vi "Attach Principal to Thing.vi"(8 "error in (no error)":errorcluster, 9 "Principal":string, 10 "Thing":string, 11 "IoT Session in":refnum<class "IoT Session.lvclass">) -> (0 "error out":errorcluster, 3 "IoT Session out":refnum<class "IoT Session.lvclass">)   [LabVIEW 2015, in "NI_AWS_IoT.lvlib" / "IoT Session.lvclass"]
uses:
  IoT Session.lvclass
  Core/HTTP Request/Request Options.ctl
  Core/HTTP Request/Name Value Pair.ctl
  Core/HTTP Request/Region handling.ctl
  Core/HTTP Request/URL formatting.ctl
  Core/HTTP Request/HTTP Request.lvclass
panel:
  # "(an example 'Principal' value is a Certificate ARN)"
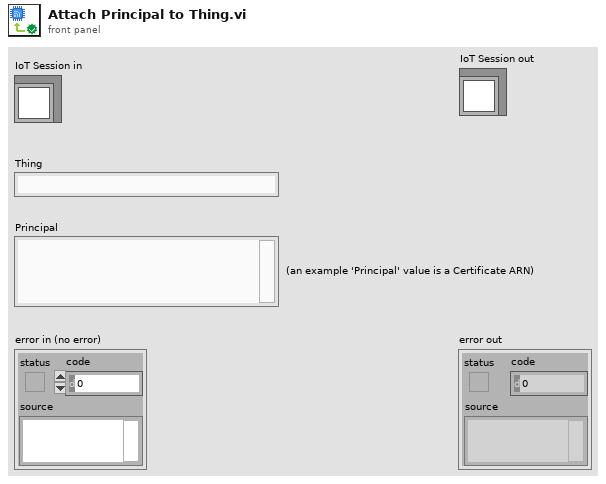
[diagram p1: front panel]
types:
  T1 = typedef "NI_AWS_Core.lvlib/HTTP Request.lvclass/Name Value Pair.ctl" = cluster{"name":string, "value":string}
  T2 = typedef "NI_AWS_Core.lvlib/HTTP Request.lvclass/Request Options.ctl" = cluster{"request headers":T1[], "request parameters":T1[], "request body":string, "region handling":T3, "URL formatting":T4}
  T3 = typedef "NI_AWS_Core.lvlib/HTTP Request.lvclass/Region handling.ctl" = enum16{"use region everywhere", "use region (authentication only)", "use region (URL only)", "ignore region everwhere"}
  T4 = typedef "NI_AWS_Core.lvlib/HTTP Request.lvclass/URL formatting.ctl" = enum16{"region-", "region."}
  T5 = typedef "NI_AWS_Core.lvlib/HTTP Request.lvclass/Response.ctl" = cluster{"Headers":string, "Body":string}
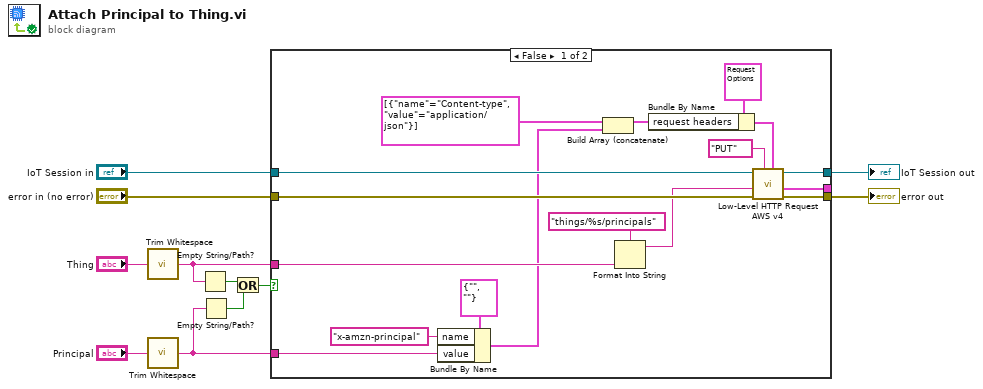
[diagram p0: block diagram]
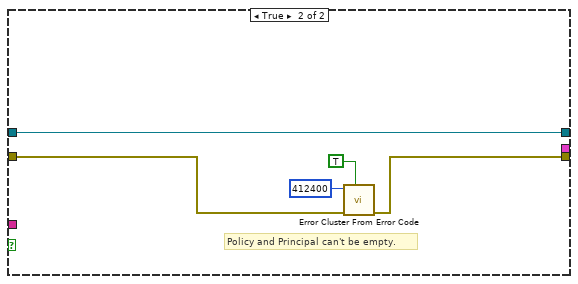
[diagram p2: hidden frame]
diagram:
  n1 = call <vilib>:"Trim Whitespace.vi"("string"="Thing") -> ("trimmed string"=w5:string)  [unwired: 1 in]
  n2 = call <vilib>:"Trim Whitespace.vi"("string"="Principal") -> ("trimmed string"=w4:string)  [unwired: 1 in]
  n3 = Empty String/Path?(string/path=w5) -> (empty?=w3:bool)
  n4 = Empty String/Path?(string/path=w4) -> (empty?=w2:bool)
  n5 = Or(x=w3, y=w2) -> (x .or. y?=w1:bool)
  n6 = case shown="False" w1 {
    tunnel: "error in (no error)" -> [w28 w33]
    tunnel: [w27 w32] -> w10
    tunnel: [w26 w30] -> w9
    tunnel: w4 -> [w15 _]
    tunnel: "IoT Session in" -> [w25 w30]
    tunnel: w5 -> [w24 _]
    tunnel: [w12 _] -> _
    frame False {
      n7 = Bundle By Name(cluster=T1 {"name"="", "value"=""} ("Cluster"), "name"="x-amzn-principal", "value"=w15) -> (w14:T1)
      n8 = Build Array (concatenate)(T1[] [{"name"="Content-type", "value"="application/json"}] ("request headers"), w14) -> (w17:T1[])
      n9 = Format Into String(format string="things/%s/principals", w24) -> (resulting string=w21:string)  [unwired: 2 in, 1 out]
      n10 = Bundle By Name(cluster=T2 {"request headers"=[], "request parameters"=[], "request body"="", "region handling"=enum."use region everywhere", "URL formatting"=enum."region."} ("Request Options"), "request headers"=w17) -> (w19:T2)
      n11 = call "Low-Level HTTP Request AWS v4.vi"("Request Options"=w19, "HTTP-Verb"="PUT", "error in (no error)"=w28, "URL Suffix"=w21, "AWS Core in"=w25) -> ("error out"=w27:errorcluster, "Response"=w12:T5, "AWS Core out"=w26:refnum<class "IoT Session.lvclass">)  [unwired: 3 in, 1 out]
    }
    frame True {
      # "Policy and Principal can't be empty."
      n12 = call <vilib>:"Error Cluster From Error Code.vi"("show call chain? (False)"=TRUE, "error in (no error)"=w33, "error code (0)"=412400) -> ("error out"=w32:errorcluster)  [unwired: 6 in]
    }
  }
  "error out" <- w10
  "IoT Session out" <- w9
